vi "main.vi"() -> ()   [LabVIEW 2018, in "Demo.lvclass"]
uses:
  Demo.lvclass
  YoutuberDownloader Class/YoutuberDownloader.lvclass
  YoutubeCacheProxy Class/YoutubeCacheProxy.lvclass
  C:/Users/fflores/Documents/LabVIEW-Open-Projects/LabIVEW OOP Design Patterns/Proxy Pattern/ThirdPartyYoutubeLib Class/ThirdPartyYoutubeLib.lvclass
  ConsoleOut/Print Options.ctl
  ThirdPartyYoutubeClass Class/ThirdPartyYoutubeClass.lvclass
  YoutuberDownloader Class/YoutuberDownloader.lvclass/YoutuberDownloader.ctl
panel:
  out "error out":errorcluster
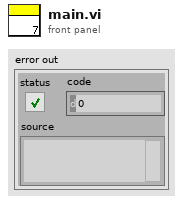
[diagram p1: front panel]
types:
  T1 = typedef "Print Options.ctl" = enum16{"Create", "Get Reference", "Print", "Print Header", "Close"}
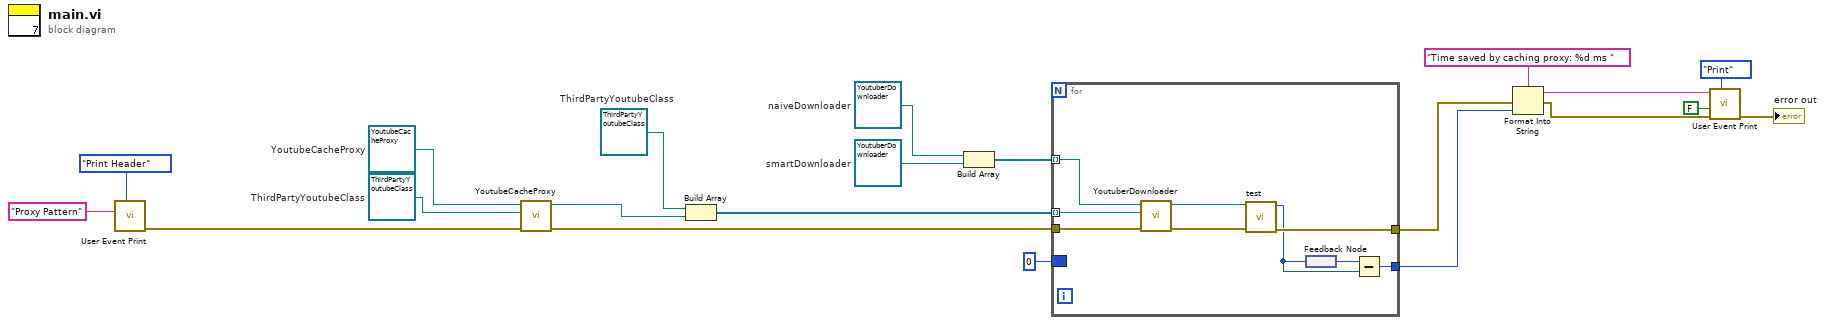
[diagram p0: block diagram]
diagram:
  w15 = refnum<class "ThirdPartyYoutubeClass.lvclass"> refnum  # ThirdPartyYoutubeClass
  w20 = refnum<class "ThirdPartyYoutubeClass.lvclass"> refnum  # ThirdPartyYoutubeClass
  w21 = refnum<class "YoutubeCacheProxy.lvclass"> refnum  # YoutubeCacheProxy
  w10 = refnum<class "YoutuberDownloader.lvclass"> refnum  # smartDownloader
  w11 = refnum<class "YoutuberDownloader.lvclass"> refnum  # naiveDownloader
  n1 = call "User Event Print.vi"("Options"=Print_Options."Print Header", "String to Print"="Proxy Pattern") -> ("error out"=w4:errorcluster)  [unwired: 8 in, 1 out]
  n2 = call "YoutubeCacheProxy.vi"("error in (no error)"=w4, "ThirdPartyYoutubeLib.lvclass"=w15, "YoutubeCacheProxy in"=w21) -> ("error out"=w3:errorcluster, "YoutubeCacheProxy out"=w9:refnum<class "YoutubeCacheProxy.lvclass">)  [unwired: 7 in]
  n3 = Build Array(w20, w9) -> (w7:refnum<class "ThirdPartyYoutubeLib.lvclass">[])
  n4 = Build Array(w11, w10) -> (w8:refnum<class "YoutuberDownloader.lvclass">[])
  n5 = for {
    tunnel: w8 -> [w29] mode=indexing
    tunnel: w7 -> [w28] mode=indexing
    border: u32 0 ("estimatedTime") -> [_]
    tunnel: [w27] -> w6
    tunnel: w3 -> [w25]
    tunnel: [w23] -> w2
    n6 = call "YoutuberDownloader.vi"("error in (no error)"=w25, "ThirdPartyYoutubeLib.lvclass"=w28, "YoutuberDownloader in"=w29) -> ("error out"=w24:errorcluster, "YoutuberDownloader out"=w30:refnum<class "YoutuberDownloader.lvclass">)  [unwired: 7 in]
    n7 = call "test.vi"("error in (no error)"=w24, "YoutuberDownloader"=w30) -> ("error out"=w23:errorcluster, "estimatedTime"=w22:u32)  [unwired: 8 in]
    n8 = feedback-in #1(w22) -> ()
    n9 = feedback #1() -> (w26:u32)
    n10 = Subtract(x=w26, y=w22) -> (x-y=w27:u32)
  }
  n11 = Format Into String(format string="Time saved by caching proxy: %d ms ", error in=w2, w6) -> (resulting string=w18:string, error out=w17:errorcluster)  [unwired: 1 in]
  n12 = call "User Event Print.vi"("Options"=Print_Options."Print", "error in (no error)"=w17, "add EOL? (T)"=FALSE, "String to Print"=w18) -> ("error out"=→"error out":errorcluster)  [unwired: 6 in, 1 out]
